vi "Pressure Limit Checker.vi"(0 "Pressure\nLimit\nTripped X":refnum<vi>, 1 "Pressure (mTorr) X":refnum<vi>, 2 "Pressure Limit":refnum<vi>, 3 "Stop / Start Reactor X":refnum<vi>, 4 "Current Cycle Reactor X":refnum<vi>, 5 "Error Trip Cycle X":refnum<vi>, 6 "System Queue":refnum<vi>, 7 "Error Trip Time X":refnum<vi>, 8 "System JSON Queue":refnum<vi>, 9 "Reactor Number":i32, 10 "Reactor Name":string, 11 "Stop Program":refnum<vi>) -> ()   [LabVIEW 2022 SP3]
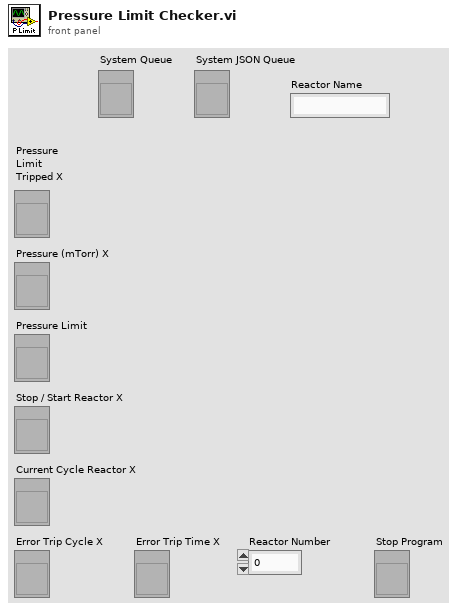
[diagram p1: front panel]
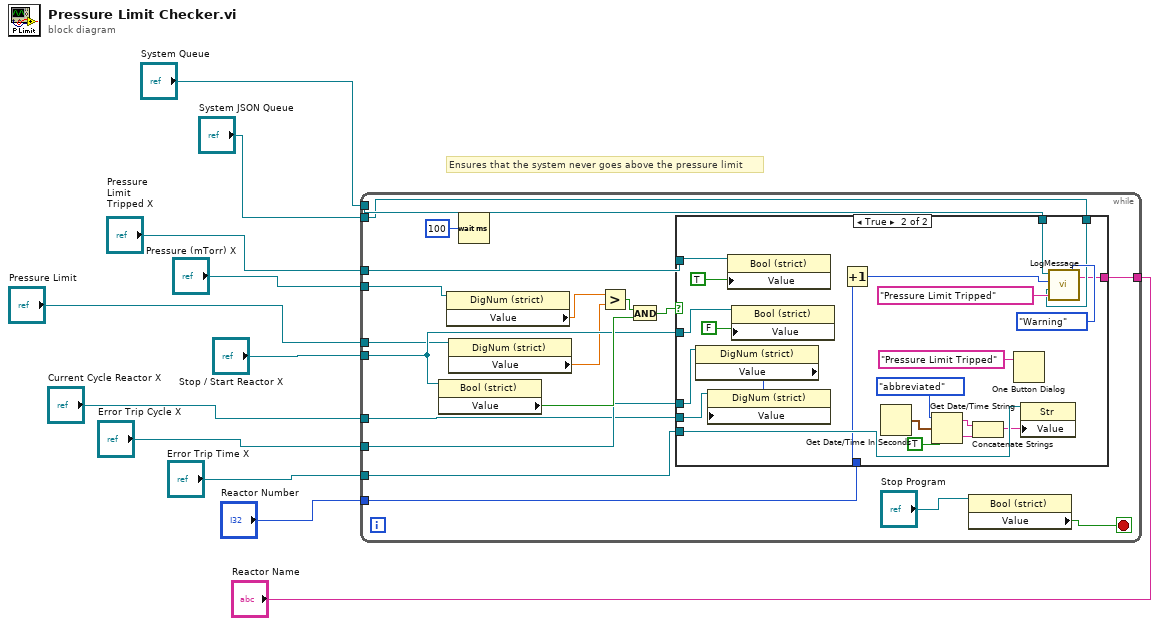
[diagram p0: block diagram]
diagram:
  # "Ensures that the system never goes above the pressure limit"
  n1 = while {
    tunnel: "Pressure (mTorr) X" -> [w30]
    tunnel: "Error Trip Cycle X" -> [w25]
    tunnel: "Current Cycle Reactor X" -> [w24]
    tunnel: "Error Trip Time X" -> [w23]
    tunnel: "Stop / Start Reactor X" -> [w22]
    tunnel: "Pressure\nLimit\nTripped X" -> [w21]
    tunnel: "Reactor Number" -> [w20]
    tunnel: "System Queue" -> [w16]
    tunnel: "System JSON Queue" -> [w15]
    tunnel: "Pressure Limit" -> [w13]
    tunnel: "Reactor Name" -> [w12]
    stop <- w18 stop-if-true
    n2 = property class="Bool (strict)"(reference=w22) -> ("Value"=w26:bool)  [unwired: 1 in, 2 out]
    n3 = property class="DigNum (strict)"(reference=w30) -> ("Value"=w27:dbl)  [unwired: 1 in, 2 out]
    n4 = property class="DigNum (strict)"(reference=w13) -> ("Value"=w14:dbl)  [unwired: 1 in, 2 out]
    n5 = Wait (ms)(milliseconds to wait=u32 100) -> ()  [unwired: 1 out]
    n6 = Greater?(x=w27, y=w14) -> (0:w29:bool)
    n7 = And(x=w29, y=w26) -> (x .and. y?=w28:bool)
    n8 = case shown="True" w28 {
      tunnel: w25 -> [_ w46]
      tunnel: w24 -> [_ w44]
      tunnel: w23 -> [_ w43]
      tunnel: w22 -> [_ w41]
      tunnel: w21 -> [_ w38]
      tunnel: w20 -> [_ w37]
      tunnel: w16 -> [_ w33]
      tunnel: w15 -> [_ w32]
      tunnel: w12 -> [_ w31]
      frame False {
      }
      frame True {
        n9 = property class="DigNum (strict)"(reference=w46) -> ("Value"=w45:i32)  [unwired: 1 in, 2 out]
        n10 = property class="DigNum (strict)"(reference=w44, "Value"=w45) -> ()  [unwired: 1 in, 2 out]
        n11 = property class="Bool (strict)"(reference=w38, "Value"=TRUE ("Pressure\nLimit\nTripped")) -> ()  [unwired: 1 in, 2 out]
        n12 = property class="Bool (strict)"(reference=w41, "Value"=FALSE ("Start/Stop Run")) -> ()  [unwired: 1 in, 2 out]
        n13 = Increment(x=w37) -> (x+1=w35:i32)
        n14 = Get Date/Time In Seconds() -> (seconds since 1Jan1904=w47:timestamp)
        n15 = Get Date/Time String(date format (0)=enum16{"short", "long", "abbreviated"}."abbreviated", seconds (now)=w47, want seconds? (F)=TRUE) -> (date string=w51:string, time string=w50:string)
        n16 = Concatenate Strings(w51, w50) -> (w42:string)
        n17 = One Button Dialog(message="Pressure Limit Tripped") -> ()  [unwired: 1 in, 1 out]
        n18 = property class="Str"(reference=w43, "Value"=w42) -> ()  [unwired: 1 in, 2 out]
        n19 = call "LogMessage.vi"("Type"=enum16{"Locks", "Warning"}."Warning", "Reactor Name"=w31, "Log Entry"="Pressure Limit Tripped", "System JSON Queue"=w32, "ID Number"=w35, "System Queue"=w33) -> ()
      }
    }
    n20 = property class="Bool (strict)"(reference="Stop Program") -> ("Value"=w18:bool)  [unwired: 1 in, 2 out]
  }
